vi "GCMPlugin_GetVI.vi"(8 "error in (no error)":errorcluster, 11 "_LVCMPlugin in":refnum<class "GCMPlugin.lvclass">) -> (0 "error out":errorcluster, 2 "VI":refnum<vi>, 3 "_LVCMPlugin out":refnum<class "GCMPlugin.lvclass">)   [LabVIEW 2014, in "GCMPlugin.lvclass"]
uses:
  GCMPlugin/GCMPlugin.lvclass
  GCMPlugin/GCMPlugin.lvclass/GCMPlugin.ctl
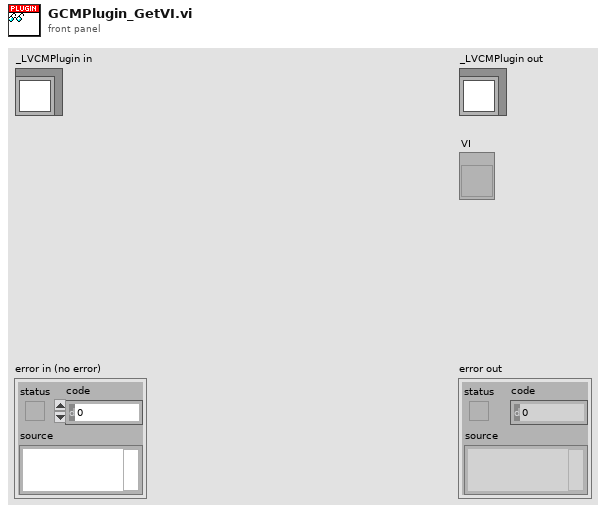
[diagram p1: front panel]
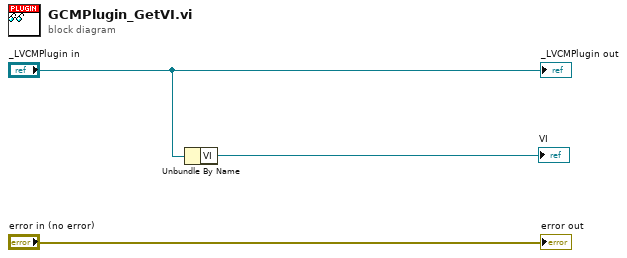
[diagram p0: block diagram]
diagram:
  n1 = Unbundle By Name("_LVCMPlugin in") -> ("VI"=→"VI":refnum<vi>)
  "error out" <- "error in (no error)"
  "_LVCMPlugin out" <- "_LVCMPlugin in"
